vi "HIOKI PW3390 Conf CT9920.vi"(0 "VISA Resource":refnum<visa-resource-name>, 1 "Set/Query (F: Set)":bool, 2 "CH (1)":i32=1 min=1 max=4, 9 "Sensor (1: 1mV/A)":T1(ring)=enum."1mV/A", 11 "error in (no error)":errorcluster, 12 "OPC query (T: ON)":bool=TRUE, 13 "Error Out (F: Off)":bool) -> (4 "VISA Resource out":refnum<visa-resource-name>, 10 "Sensor out":T1(ring)=enum."1mV/A", 15 "error out":errorcluster)   [LabVIEW 2009]
doc: "Sets and reads the setting of current sensor for CT9920.\n\nSet/Query\n Set: Send the setting commands for the device.\n Query: Query the setting of the device.\n\nSensor\n Sets the current sensor setting for CT9920."
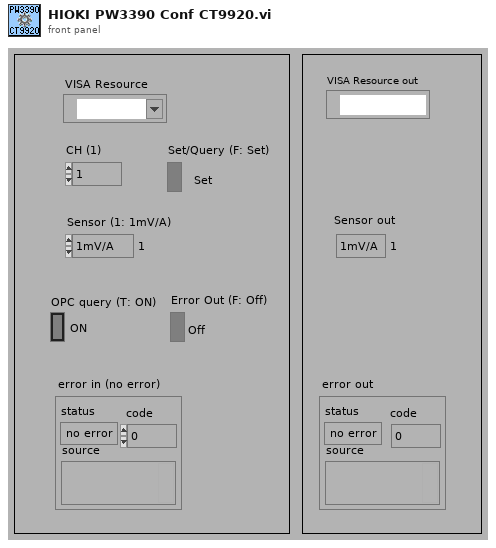
[diagram p1: front panel]
types:
  T1 = enum16{"100uV/A", "1mV/A", "10mV/A", "100mV/A", "CT7642", "CT7742", "CT7044", "CT7045", "CT7046"}
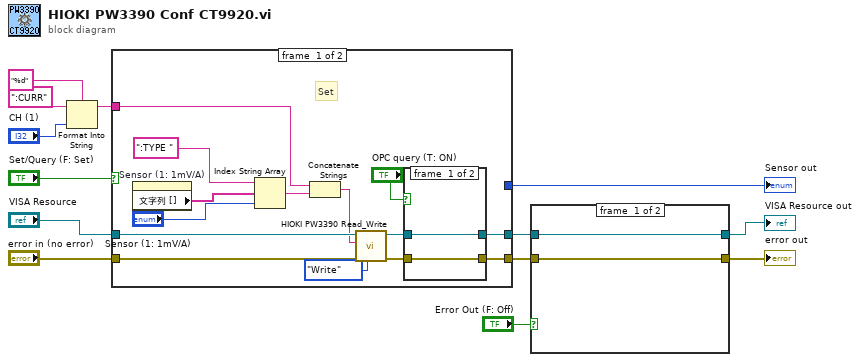
[diagram p0: block diagram]
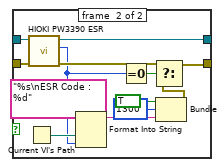
[diagram p2: hidden frame]
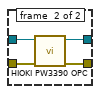
[diagram p3: hidden frame]
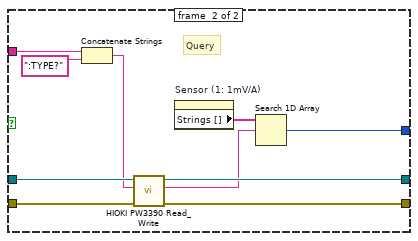
[diagram p4: hidden frame]
diagram:
  n1 = Format Into String(format string="%d", initial string=":CURR", "CH (1)") -> (resulting string=w8:string)  [unwired: 1 in, 1 out]
  n2 = case shown="FALSE" "Set/Query (F: Set)" {
    tunnel: "error in (no error)" -> [w23 w40]
    tunnel: [w17 w37] -> w6
    tunnel: "VISA Resource" -> [w24 w41]
    tunnel: [w18 w38] -> w5
    tunnel: w8 -> [w16 w42]
    tunnel: [_ w34] -> w1
    frame #0 {
      # "Set"
      n3 = property on="Sensor (1: 1mV/A)" class="Enum （指定）"() -> ("文字列 []"=w26:string[])  [unwired: 2 in, 2 out]
      n4 = Index String Array(1:"Sensor (1: 1mV/A)", 2:w26, 3:":TYPE ") -> (0:w15:string)
      n5 = Concatenate Strings(w16, w15) -> (w14:string)
      n6 = call <instrlib>:"HIOKI PW3390 Read_Write.vi"("Read/Write"=enum16{"Read", "Write"}."Write", "error in (no error)"=w23, "data in"=w14, "VISA Resource"=w24) -> ("error out"=w19:errorcluster, "VISA Resource out"=w20:refnum<visa-resource-name>)  [unwired: 5 in, 1 out]
      n7 = case shown="TRUE" "OPC query (T: ON)" {
        tunnel: [w29 w33] -> w18
        tunnel: [w28 w32] -> w17
        tunnel: w20 -> [w29 w31]
        tunnel: w19 -> [w28 w30]
        frame #0 {
        }
        frame #1 {
          n8 = call <instrlib>:"HIOKI PW3390 OPC.vi"("error in (no error)"=w30, "VISA Resource"=w31) -> ("error out"=w32:errorcluster, "VISA Resource out"=w33:refnum<visa-resource-name>)  [unwired: 7 in, 1 out]
        }
      }
    }
    frame #1 {
      # "Query"
      n9 = Concatenate Strings(w42, ":TYPE?") -> (w39:string)
      n10 = call <instrlib>:"HIOKI PW3390 Read_Write.vi"("error in (no error)"=w40, "data in"=w39, "VISA Resource"=w41) -> ("error out"=w37:errorcluster, "data out"=w35:string, "VISA Resource out"=w38:refnum<visa-resource-name>)  [unwired: 6 in]
      n11 = property on="Sensor (1: 1mV/A)" class="Enum （指定）"() -> ("Strings []"=w36:string[])  [unwired: 2 in, 2 out]
      n12 = Search 1D Array(1D array=w36, element=w35) -> (index of element=w34:i32)  [unwired: 1 in]
    }
  }
  "Sensor out" <- w1
  n13 = case shown="TRUE" "Error Out (F: Off)" {
    tunnel: w5 -> [w45 w58]
    tunnel: w6 -> [w44 w57]
    tunnel: [w44 w47] -> w4
    tunnel: [w45 w56] -> w2
    frame #0 {
    }
    frame #1 {
      n14 = Current VI's Path() -> (path=w54:path)
      n15 = call <instrlib>:"HIOKI PW3390 ESR.vi"("error in (no error)"=w57, "VISA Resource"=w58) -> ("error out"=w48:errorcluster, "Output Value"=w46:u8, "VISA Resource out"=w56:refnum<visa-resource-name>)  [unwired: 6 in, 1 out]
      n16 = Format Into String(format string="%s\nESR Code : %d", w54, w46) -> (resulting string=w50:string)  [unwired: 2 in, 1 out]
      n17 = Equal To 0?(x=w46) -> (x = 0?=w55:bool)
      n18 = Bundle("status"=TRUE, "code"=1300, w50) -> (w49:cluster{"status":bool, "code":i32, string})  [unwired: 1 in]
      n19 = Select(t=w48, s=w55, f=w49) -> (s? t:f=w47:errorcluster)
    }
  }
  "error out" <- w4
  "VISA Resource out" <- w2
